vi "SEK2020v1VI11ColocarTubo.vi"(9 "Parâmetros":T1={"Azul Max EV3 Cor"=17, "Azul Min EV3 Cor"=0, "Verde Max EV3 Cor"=6, "Verde Min EV3 Cor"=0, "Vermelho Max Ev3 Cor"=0, "Vermelho Min EV3 Cor"=0, "Chão EV3 Cor"=0.0, "Branco Max EV3 Cor"=0.0, "Branco Min EV3 Cor"=0.0, "Preto Max EV3 Cor"=0.0, "Preto Min EV3 Cor"=0.0, "Distância Tubulação"=0.0, "Distância Frontal"=0.0, "Amarelo Max EV3 Cor"=0.0, "Amarelo Min EV3 Cor"=0.0, "Distância Lateral"=0.0, "90°"=0.0, "180°"=0.0, "Seguidor de Linha"=0.0}, 10 "NXT/EV3":T2) -> (2 "NXT/EV3 2":T2)   [LabVIEW 2016]
uses:
  <vilib>/NXT/Subs/LVHSConnector.ctl
  <vilib>/NXT/LegoClasses/BrickReference/BrickReference.lvclass
  <vilib>/NXT/Block Support/NXT_OutputPort.ctl
  <vilib>/NXT/NXTIO Xnodes/NXTIONodeSubVIs/NXTMoveMotors.vi
  <vilib>/NXT/NXTIO Xnodes/NXTIONodeSubVIs/NXTStopMotors.vi
  <vilib>/NXT/Dual Mode Library/Waits/Wait_Num.vi
  <vilib>/NXT/NXTIO Xnodes/AddressXNode/NXTIOAddress.xnode
  <vilib>/NXT/NXTIO Xnodes/NXTIOXNode/NXTIO.xnode
panel:
  # "Sensor EV3 Cor"
  # "Sensor Ultrassônico"
  # "Sensor Giroscópio"
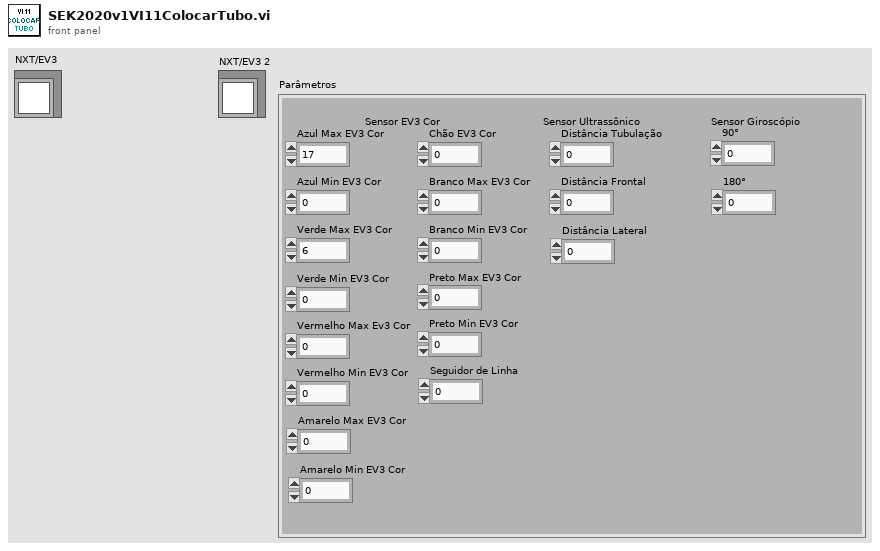
[diagram p1: front panel]
types:
  T1 = cluster{"Azul Max EV3 Cor":i32, "Azul Min EV3 Cor":i32, "Verde Max EV3 Cor":i32, "Verde Min EV3 Cor":i32, "Vermelho Max Ev3 Cor":i32, "Vermelho Min EV3 Cor":i32, "Chão EV3 Cor":sgl, "Branco Max EV3 Cor":sgl, "Branco Min EV3 Cor":sgl, "Preto Max EV3 Cor":sgl, "Preto Min EV3 Cor":sgl, "Distância Tubulação":sgl, "Distância Frontal":sgl, "Amarelo Max EV3 Cor":dbl, "Amarelo Min EV3 Cor":dbl, "Distância Lateral":sgl, "90°":sgl, "180°":sgl, "Seguidor de Linha":dbl}
  T2 = typedef "LVHSConnector.ctl" = refnum<class "BrickReference.lvclass">
  T3 = typedef "NXT_OutputPort.ctl" = u8
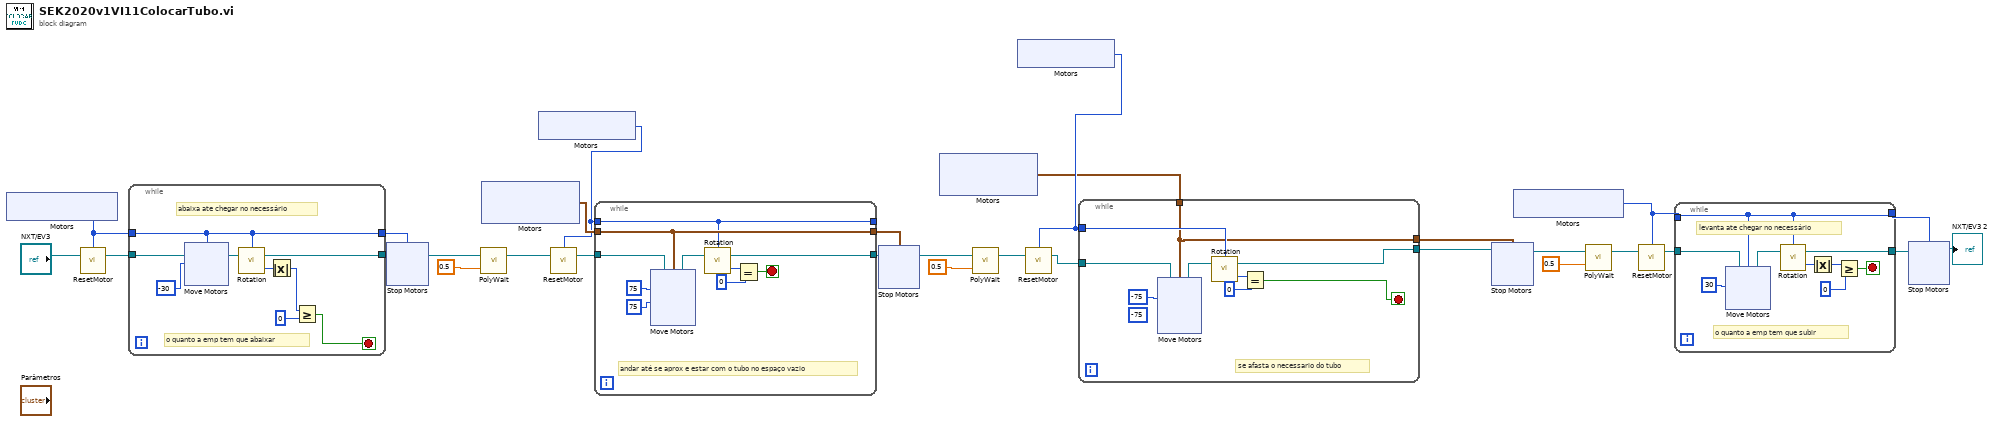
[diagram p0: block diagram]
diagram:
  n1 = xnode "Motors"() -> ("Motor"=w28:T3)
  n2 = call <vilib>:"ResetMotor.vi"("NXT/EV3"="NXT/EV3", "Port (All Ports)"=w28) -> ("NXT/EV3"=w29:T2)  [unwired: 2 in]
  n3 = while {
    tunnel: w29 -> [w38]
    tunnel: w28 -> [w36]
    tunnel: [w36] -> w27
    tunnel: [w34] -> w24
    stop <- w31 stop-if-true
    # "abaixa ate chegar no necessário"
    # "o quanto a emp tem que abaixar"
    n4 = xnode "Move Motors"("Power/Speed 1"=i8 -30, "Motors"=w36, "NXT/EV3"=w38) -> ("NXT/EV3"=w35:T2)
    n5 = call <vilib>:"Rotation.vi"("NXT/EV3"=w35, "Port (Port A)"=w36) -> ("Angle of Rotation"=w33:i32, "NXT/EV3"=w34:T2)  [unwired: 1 in]
    n6 = Absolute Value(x=w33) -> (abs(x)=w32:i32)
    n7 = Greater Or Equal?(x=w32, y=0) -> (x >= y?=w31:bool)
  }
  n8 = xnode "Stop Motors"("Motors"=w27, "NXT/EV3"=w24) -> ("NXT/EV3"=w20:T2)
  n9 = call-poly <vilib>:"PolyWait.vi"("Time (1 sec)"=sgl 0.5, "NXT/EV3"=w20) -> ("NXT/EV3"=w19:T2)  [unwired: 2 in]
  n10 = xnode "Motors"() -> ("Motor"=w26:cluster{"Port":T3, "Port":T3})
  n11 = xnode "Motors"() -> ("Motor"=w14:T3)
  n12 = call <vilib>:"ResetMotor.vi"("NXT/EV3"=w19, "Port (All Ports)"=w14) -> ("NXT/EV3"=w25:T2)  [unwired: 2 in]
  n13 = while {
    tunnel: w26 -> [w52]
    tunnel: [w48] -> w23
    tunnel: [w52] -> w22
    tunnel: w25 -> [w50]
    tunnel: w14 -> [w47]
    tunnel: [w47] -> _
    stop <- w54 stop-if-true
    # "andar até se aprox e estar com o tubo no espaço vazio"
    n14 = xnode "Move Motors"("Power/Speed 2"=i8 75, "Power/Speed 1"=i8 75, "Motors"=w52, "NXT/EV3"=w50) -> ("NXT/EV3"=w49:T2)
    n15 = call <vilib>:"Rotation.vi"("NXT/EV3"=w49, "Port (Port A)"=w47) -> ("Angle of Rotation"=w55:i32, "NXT/EV3"=w48:T2)  [unwired: 1 in]
    n16 = Equal?(x=w55, y=0) -> (x = y?=w54:bool)
  }
  n17 = xnode "Stop Motors"("Motors"=w22, "NXT/EV3"=w23) -> ("NXT/EV3"=w16:T2)
  n18 = xnode "Motors"() -> ("Motor"=w11:cluster{"Port":T3, "Port":T3})
  n19 = call-poly <vilib>:"PolyWait.vi"("Time (1 sec)"=sgl 0.5, "NXT/EV3"=w16) -> ("NXT/EV3"=w17:T2)  [unwired: 2 in]
  n20 = xnode "Motors"() -> ("Motor"=w12:T3)
  n21 = call <vilib>:"ResetMotor.vi"("NXT/EV3"=w17, "Port (All Ports)"=w12) -> ("NXT/EV3"=w13:T2)  [unwired: 2 in]
  n22 = while {
    tunnel: w13 -> [w69]
    tunnel: w12 -> [w68]
    tunnel: w11 -> [w66]
    tunnel: [w67] -> w2
    tunnel: [w66] -> w1
    stop <- w65 stop-if-true
    (unwired) i8 -75 ("Power/Speed 2")
    # "se afasta o necessario do tubo"
    n23 = xnode "Move Motors"("Power/Speed 1"=i8 -75, "Motors"=w66, "NXT/EV3"=w69) -> ("NXT/EV3"=w70:T2)  [unwired: 1 in]
    n24 = call <vilib>:"Rotation.vi"("NXT/EV3"=w70, "Port (Port A)"=w68) -> ("Angle of Rotation"=w72:i32, "NXT/EV3"=w67:T2)  [unwired: 1 in]
    n25 = Equal?(x=w72, y=0) -> (x = y?=w65:bool)
  }
  n26 = xnode "Stop Motors"("Motors"=w1, "NXT/EV3"=w2) -> ("NXT/EV3"=w4:T2)
  n27 = xnode "Motors"() -> ("Motor"=w9:T3)
  n28 = call-poly <vilib>:"PolyWait.vi"("Time (1 sec)"=sgl 0.5, "NXT/EV3"=w4) -> ("NXT/EV3"=w5:T2)  [unwired: 2 in]
  n29 = call <vilib>:"ResetMotor.vi"("NXT/EV3"=w5, "Port (All Ports)"=w9) -> ("NXT/EV3"=w10:T2)  [unwired: 2 in]
  n30 = while {
    tunnel: w10 -> [w88]
    tunnel: w9 -> [w86]
    tunnel: [w86] -> w8
    tunnel: [w84] -> w7
    stop <- w89 stop-if-true
    # "o quanto a emp tem que subir"
    # "levanta ate chegar no necessário"
    n31 = xnode "Move Motors"("Power/Speed 1"=i8 30, "Motors"=w86, "NXT/EV3"=w88) -> ("NXT/EV3"=w85:T2)
    n32 = call <vilib>:"Rotation.vi"("NXT/EV3"=w85, "Port (Port A)"=w86) -> ("Angle of Rotation"=w83:i32, "NXT/EV3"=w84:T2)  [unwired: 1 in]
    n33 = Absolute Value(x=w83) -> (abs(x)=w82:i32)
    n34 = Greater Or Equal?(x=w82, y=0) -> (x >= y?=w89:bool)
  }
  n35 = xnode "Stop Motors"("Motors"=w8, "NXT/EV3"=w7) -> ("NXT/EV3"=→"NXT/EV3 2":T2)
